vi "Pre-Init.vi"(8 "error in (no error)":errorcluster, 11 "DAQmx Synthesizer in":refnum<class "DAQmx Synthesizer.lvclass">) -> (0 "error out":errorcluster, 3 "DAQmx Synthesizer out":refnum<class "DAQmx Synthesizer.lvclass">)   [LabVIEW 2019, in "DAQmx Synthesizer.lvclass"]
uses:
  DAQmx Synthesizer.lvclass
  Instruments/Pulse Driver/Pulse Driver.lvclass
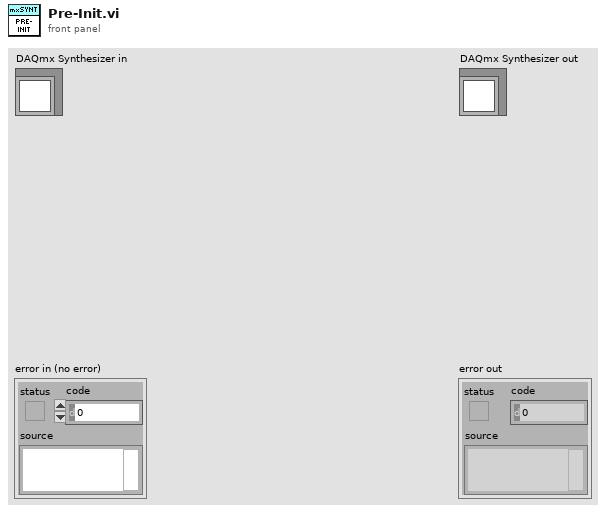
[diagram p1: front panel]
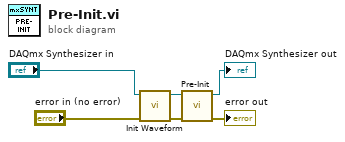
[diagram p0: block diagram]
diagram:
  n1 = call-dynamic "Init Waveform.vi"("error in (no error)"="error in (no error)", "DAQmx Synthesizer in"="DAQmx Synthesizer in") -> ("error out"=w1:errorcluster, "DAQmx Synthesizer out"=w3:refnum<class "DAQmx Synthesizer.lvclass">)  [unwired: 8 in]
  n2 = call-parent "Pre-Init.vi"("error in (no error)"=w1, "Pulse Driver in"=w3) -> ("error out"=→"error out":errorcluster, "Pulse Driver out"=→"DAQmx Synthesizer out":refnum<class "DAQmx Synthesizer.lvclass">)  [unwired: 8 in]
